vi "Modify NumNodes in SPI Engine.vi"(7 "VI to Code Relative Path":string="IONode\\SPIEngineSOM.vi", 8 "Error In":errorcluster, 10 "Number of Nodes":i32, 11 "Source Root Path":path=path "C:/Users/kvemishe/Downloads/TestScript") -> (0 "Error Out":errorcluster, 1 "NumCasesFound":i32, 2 "Found Object?":bool, 3 "Source Root Path Out":path=path "C:/Users/kvemishe/Downloads/IONode/DLULayer/Dequeue Cmds From Nodes.vi")   [LabVIEW 2014]
doc: "This VI scripts the deque commands VI for the IO Node Engine"
uses:
  <vilib>/Utility/traverseref.llb/TRef TravTarget.ctl
  <vilib>/Utility/traverseref.llb/VI Scripting - Traverse.lvlib
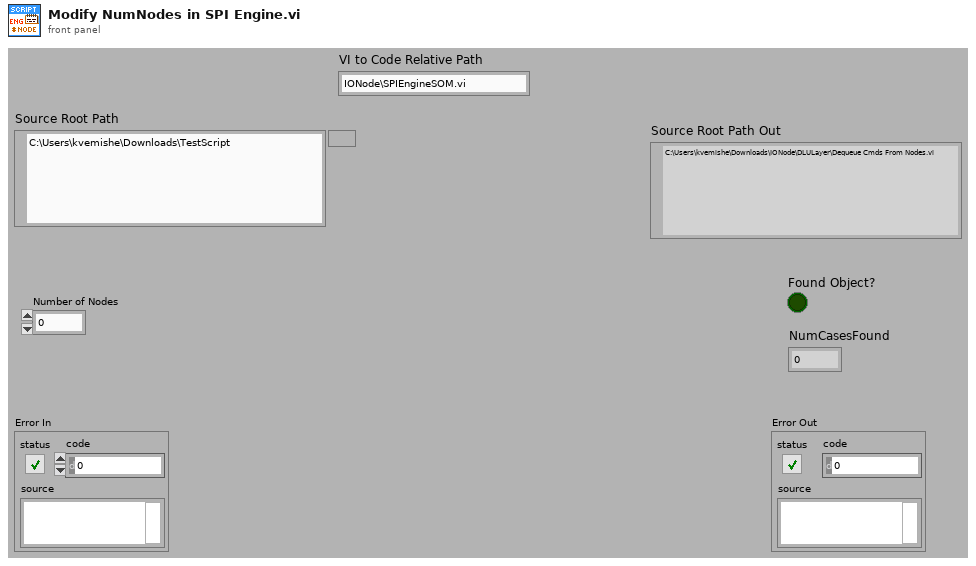
[diagram p1: front panel]
types:
  T1 = typedef "TRef TravTarget.ctl" = enum16{"FP", "BD", "Other"}
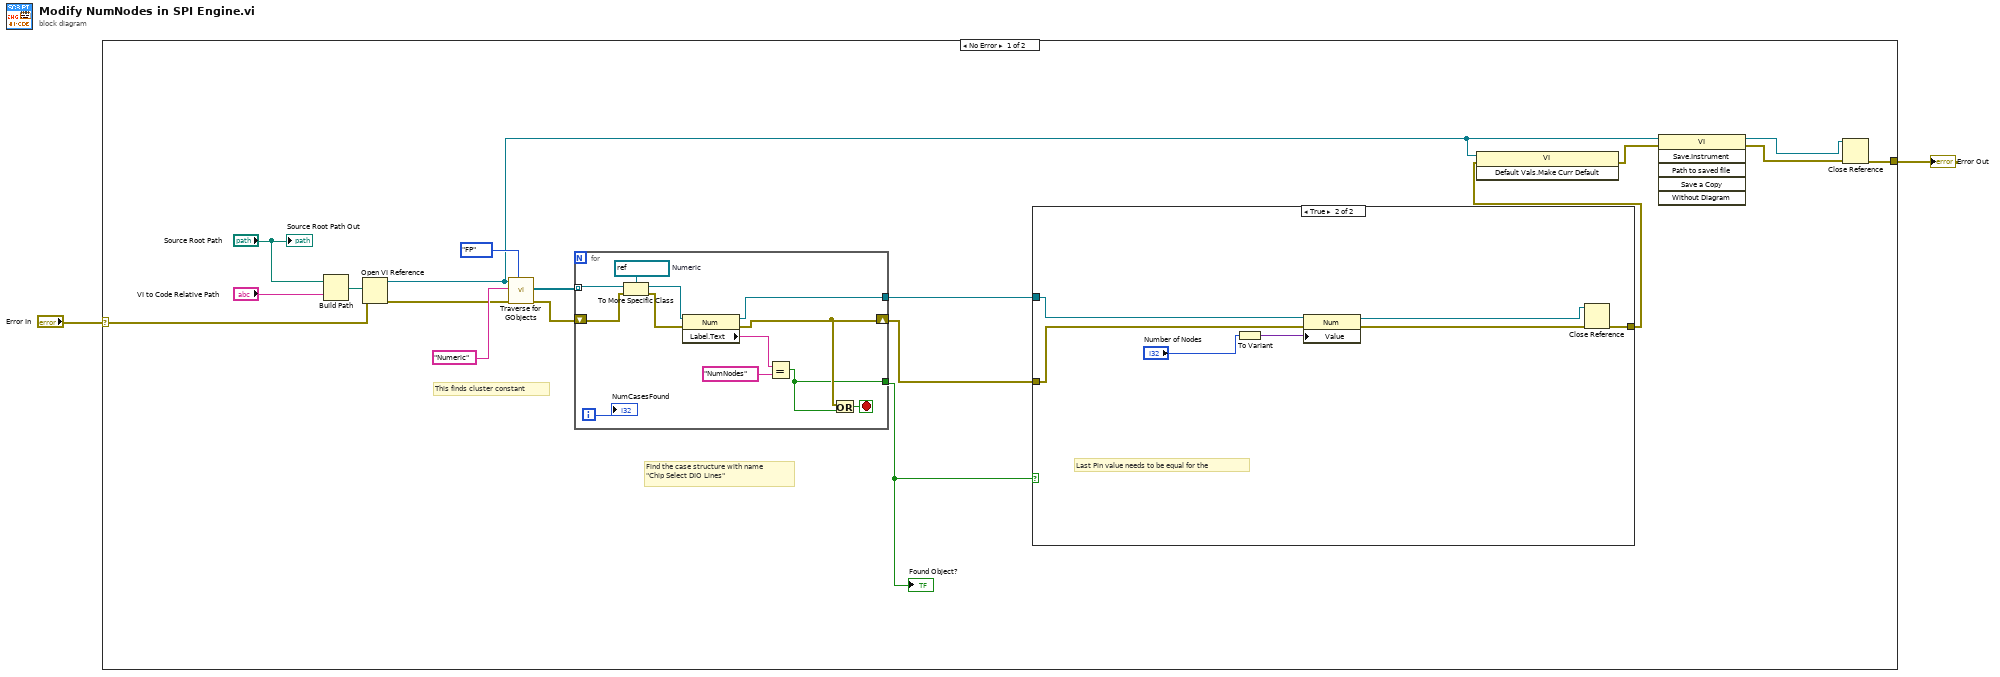
[diagram p0: block diagram]
diagram:
  n1 = case shown="No Error" "Error In" {
    selector: "Error In" -> [w13 w41]
    tunnel: [w12 w41] -> w1
    frame No Error {
      # "Find the case structure with name\n\"Chip Select DIO Lines\""
      # "This finds cluster constant"
      n2 = Build Path(base path="Source Root Path", name or relative path="VI to Code Relative Path") -> (appended path=w9:path)
      n3 = Open VI Reference(vi path=w9, error in (no error)=w13) -> (vi reference=w5:refnum<vi>, error out=w6:errorcluster)  [unwired: 4 in]
      n4 = call <vilib>:"Traverse for GObjects.vi"("Traverse Target"=TRef_TravTarget."FP", "error in (no error)"=w6, "Class Name"="Numeric", "VI Refnum"=w5) -> ("error out"=w17:errorcluster, "References"=w18:refnum<vi>[])  [unwired: 4 in, 2 out]
      n5 = for {
        tunnel: w18 -> [w40] mode=indexing
        shift-right: [w32] -> w15
        shift-left: w17 -> [w38]
        tunnel: [w31] -> w14
        tunnel: [w30] -> w16
        i -> [w29]
        stop <- w33 stop-if-true
        w39 = refnum<vi> refnum  # Numeric
        n6 = To More Specific Class(target class=w39, reference=w40, error in=w38) -> (specific class reference=w37:refnum<vi>, error out=w36:errorcluster)
        n7 = property class="Num"(reference=w37, error in=w36) -> (reference out=w30:refnum<vi>, error out=w32:errorcluster, "Label.Text"=w35:string)
        n8 = Equal?(x=w35, y="NumNodes") -> (x = y?=w31:bool)
        n9 = Or(x=w32, y=w31) -> (x .or. y?=w33:bool)
        "NumCasesFound" <- w29
      }
      "Found Object?" <- w14
      n10 = case shown="True" w14 {
        tunnel: w16 -> [_ w27]
        tunnel: w15 -> [w21 w26]
        tunnel: [w21 w23] -> w8
        frame False {
        }
        frame True {
          # "Last Pin value needs to be equal for the"
          n11 = To Variant(anything="Number of Nodes") -> (Variant=w25:variant)
          n12 = property class="Num"(reference=w27, error in=w26, "Value"=w25) -> (reference out=w22:refnum<vi>, error out=w24:errorcluster)
          n13 = Close Reference(reference=w22, error in (no error)=w24) -> (error out=w23:errorcluster)
        }
      }
      n14 = invoke class="VI" method="Default Vals.Make Curr Default"(reference=w5, error in=w8) -> (error out=w7:errorcluster)  [unwired: 1 in, 2 out]
      n15 = invoke class="VI" method="Save.Instrument"(reference=w5, error in=w7) -> (reference out=w3:refnum<vi>, error out=w4:errorcluster)  [unwired: 4 in, 4 out]
      n16 = Close Reference(reference=w3, error in (no error)=w4) -> (error out=w12:errorcluster)
      "Source Root Path Out" <- "Source Root Path"
    }
    frame Error {
    }
  }
  "Error Out" <- w1
